vi "IMU Orient Demo.vi"() -> ()   [LabVIEW 2014]
doc: "This example shows how to move a motor connected to an encoder and a wheel, and then read information about the system from an encoder.\n\nThis is an example of how to use feedback (from the encoder) to create an open loop system. If some control method was used, for example using PID, a closed loop system could be created."
uses:
  <vilib>/Rock Robotics/SystemInterfaces/i2clib/i2c_bus.ctl
  <vilib>/Platform/TimedLoop/XDataNode/timing_clust.ctl
  <vilib>/Platform/TimedLoop/XDataNode/nitl_modes.ctl
  <vilib>/Platform/TimedLoop/XDataNode/wakeup.ctl
  <vilib>/Rock Robotics/Network Tables/SD Write Number.vi
  <vilib>/platform/TimedLoop/XDataNode/XDataNode.xnode
  <vilib>/Platform/TimedLoop/XDataNode/XDNodeRunTimeDep.lvlib
panel:
  in  "Status delay":i32=30
  out "Bad result":bool
  in  "Op Mode":T1(ring)=enum."NDOF_FMC_OFF"
  in  "Earth Field (uT)":cluster{"Earth":dbl, "Tolerance":dbl}={"Earth"=51.0, "Tolerance"=5.0}
  out "Anomaly":bool
  out "Z Mag":dbl
  out "Y Mag":dbl
  out "X Mag":dbl
  in  "Read Enable":T2={"Cal Status"=TRUE, "Orientation"=TRUE, "Gyro"=FALSE, "Accelerometer"=FALSE, "Quaternion"=FALSE, "Accel Mode"=enum."Linear", "Magnetometer"=FALSE}
  in  "Calibrate?":bool
  in  "Stored Cal File":string="BNO055 Cal MC P3 11-28-2015 145653"
  out "Q Z":dbl
  out "Q Y":dbl
  out "Q X":dbl
  out "Q W":dbl
  out "GR X":dbl
  out "GR Y":dbl
  out "GR Z":dbl
  in  "Gyro Reset":bool
  out "A X":dbl
  out "A Y":dbl
  out "A Z":dbl
  out "G X":dbl(graph)
  out "G Y":dbl(graph)
  out "G Z":dbl(graph)
  out "M 2":T3
  out "A 2":T3
  out "G 2":T3
  out "S 2":T3
  out "Pitch":dbl(graph)
  out "Roll":dbl(graph)
  out "Yaw":dbl(graph)
  out "M":T3
  out "A":T3
  out "G":T3
  out "S":T3
  in  "I2C Bus":T4=enum."I2C MXP"
  in  "Period (dt in ms)":i64=20
  out "Late?":bool
  # "Magnetic Field Strength (uT)"
  # "Acceleration (mG)"
  # "Gyro Rate (Degrees per Second)"
  # "Quaternions"
  # "Cal Status @ Open"
  # "Current Cal Status"
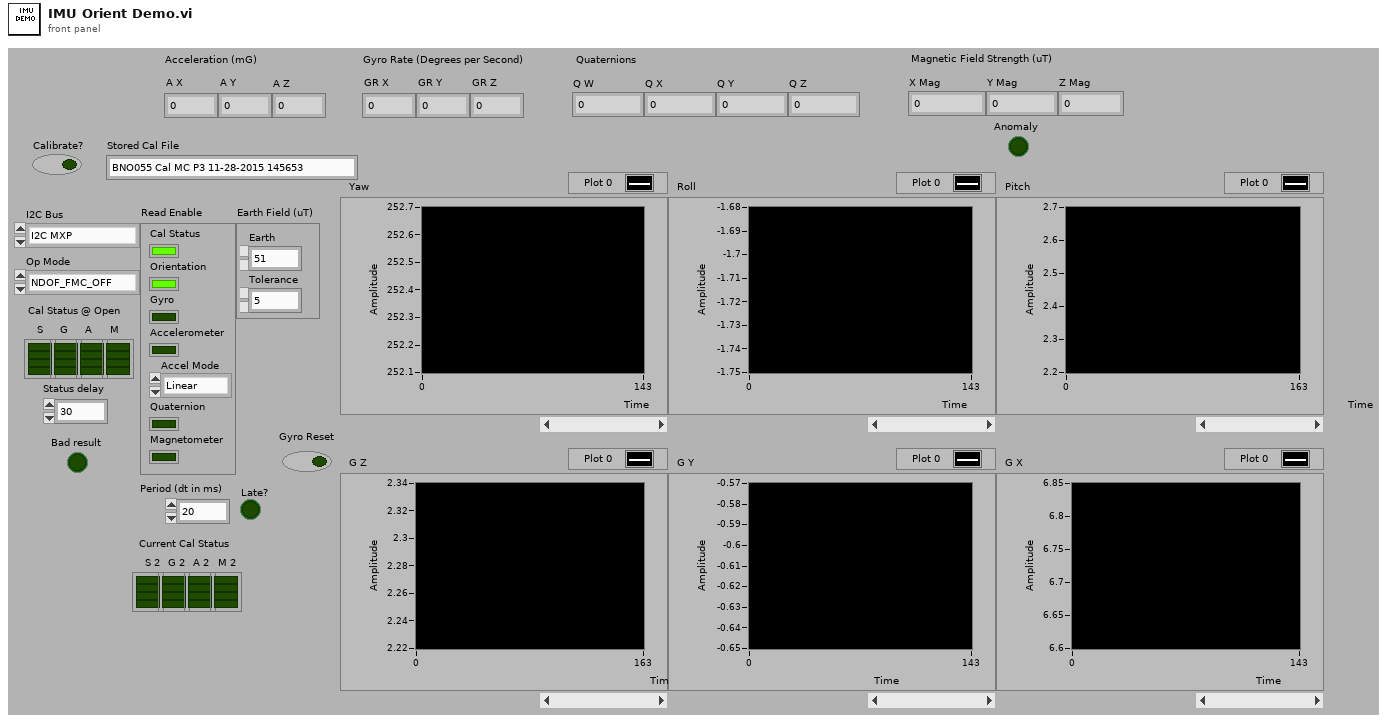
[diagram p1: front panel]
types:
  T1 = enum8{"ConfigMode", "AccOnly", "MagOnly", "GyroOnly", "AccMag", "AccGyro", "MagGyro", "AMG", "IMU", "Compass", "M4G", "NDOF_FMC_OFF", "NDOF"}
  T2 = cluster{"Cal Status":bool, "Orientation":bool, "Gyro":bool, "Accelerometer":bool, "Quaternion":bool, "Accel Mode":enum8{"Raw Data", "Linear", "Gravity"}, "Magnetometer":bool}
  T3 = cluster{"Boolean":bool, "Boolean 2":bool, "Boolean 3":bool, "Boolean 4":bool}
  T4 = typedef "i2c_bus.ctl" = enum16{"I2C On-Board", "I2C MXP", "Invalid"}
  T5 = enum32{"P0", "P1", "P2", "P3", "P4", "P5", "P6", "P7"}
  T6 = cluster{"Cluster":cluster{"[0]":bool, "[1]":bool, "[2]":bool, "[3]":bool}, "Cluster":cluster{"[0]":bool, "[1]":bool, "[2]":bool, "[3]":bool}, "Cluster":cluster{"[0]":bool, "[1]":bool, "[2]":bool, "[3]":bool}, "Cluster":cluster{"[0]":bool, "[1]":bool, "[2]":bool, "[3]":bool}}
  T7 = typedef "WPI_I2CDevRef.ctl" = cluster{"DevStatus":errorcluster, "Controller":T8, "Device Address":u8, "Handle":i32, "I2C Bus":T4}
  T8 = typedef "FPGA_TypedefDigitalModule.ctl" = enum16{"Controller 1"}
  T9 = cluster{"[0]":bool, "[1]":bool, "[2]":bool, "[3]":bool}
  T10 = typedef "XDNodeRunTimeDep.lvlib/timing_clust.ctl" = cluster{"Expected End [f-1]":u64, "Actual End [f-1]":u64, "Finished Late? [f-1]":bool, "Expected End [i-1]":u64, "Actual End [i-1]":u64, "Finished Late? [i-1]":bool, "Expected Start [i]":u64, "Actual Start [i]":u64, "Expected Start [f]":u64, "Actual Start [f]":u64, "Source Name":string, "Structure Name":string, "Period":i64, "Deadline":i64, "Offset":i64, "Start":i64, "Priority":i32, "Timeout":i32, "Mode":T11, "Wakeup Reason":T12, "Error":errorcluster, "Source Type":string, "Secondary Source Type":string, "Global End Time":u64, "Global Start Time":u64, "Frame Duration":u64, "Iteration Duration":u64, "Assigned CPU":i32, "I/O Scan Engine Mode":u32}
  T11 = typedef "XDNodeRunTimeDep.lvlib/nitl_modes.ctl" = enum32{"No Change", "Process missed periods, maintain original phase", "Discard missed periods, maintain original phase", "Process missed periods, ignore original phase", "Discard missed periods, ignore original phase"}
  T12 = typedef "XDNodeRunTimeDep.lvlib/wakeup.ctl" = enum32{"Normal", "Aborted", "Asynchronous wakeup", "Timing source error", "Timed loop error", "Timeout"}
  T13 = cluster{"Mag":cluster{"[0]":bool, "[1]":bool, "[2]":bool, "[3]":bool}, "Acc":cluster{"[0]":bool, "[1]":bool, "[2]":bool, "[3]":bool}, "Gyro":cluster{"[0]":bool, "[1]":bool, "[2]":bool, "[3]":bool}, "Sys":cluster{"[0]":bool, "[1]":bool, "[2]":bool, "[3]":bool}}
  T14 = cluster{"X Gyro":dbl, "Y Gyro":dbl, "Z Gyro":dbl, "X Rate":dbl, "Y Rate":dbl, "Z Rate":dbl}
  T15 = cluster{"X Mag":dbl, "Y Mag":dbl, "Z Mag":dbl, "Anomaly":bool}
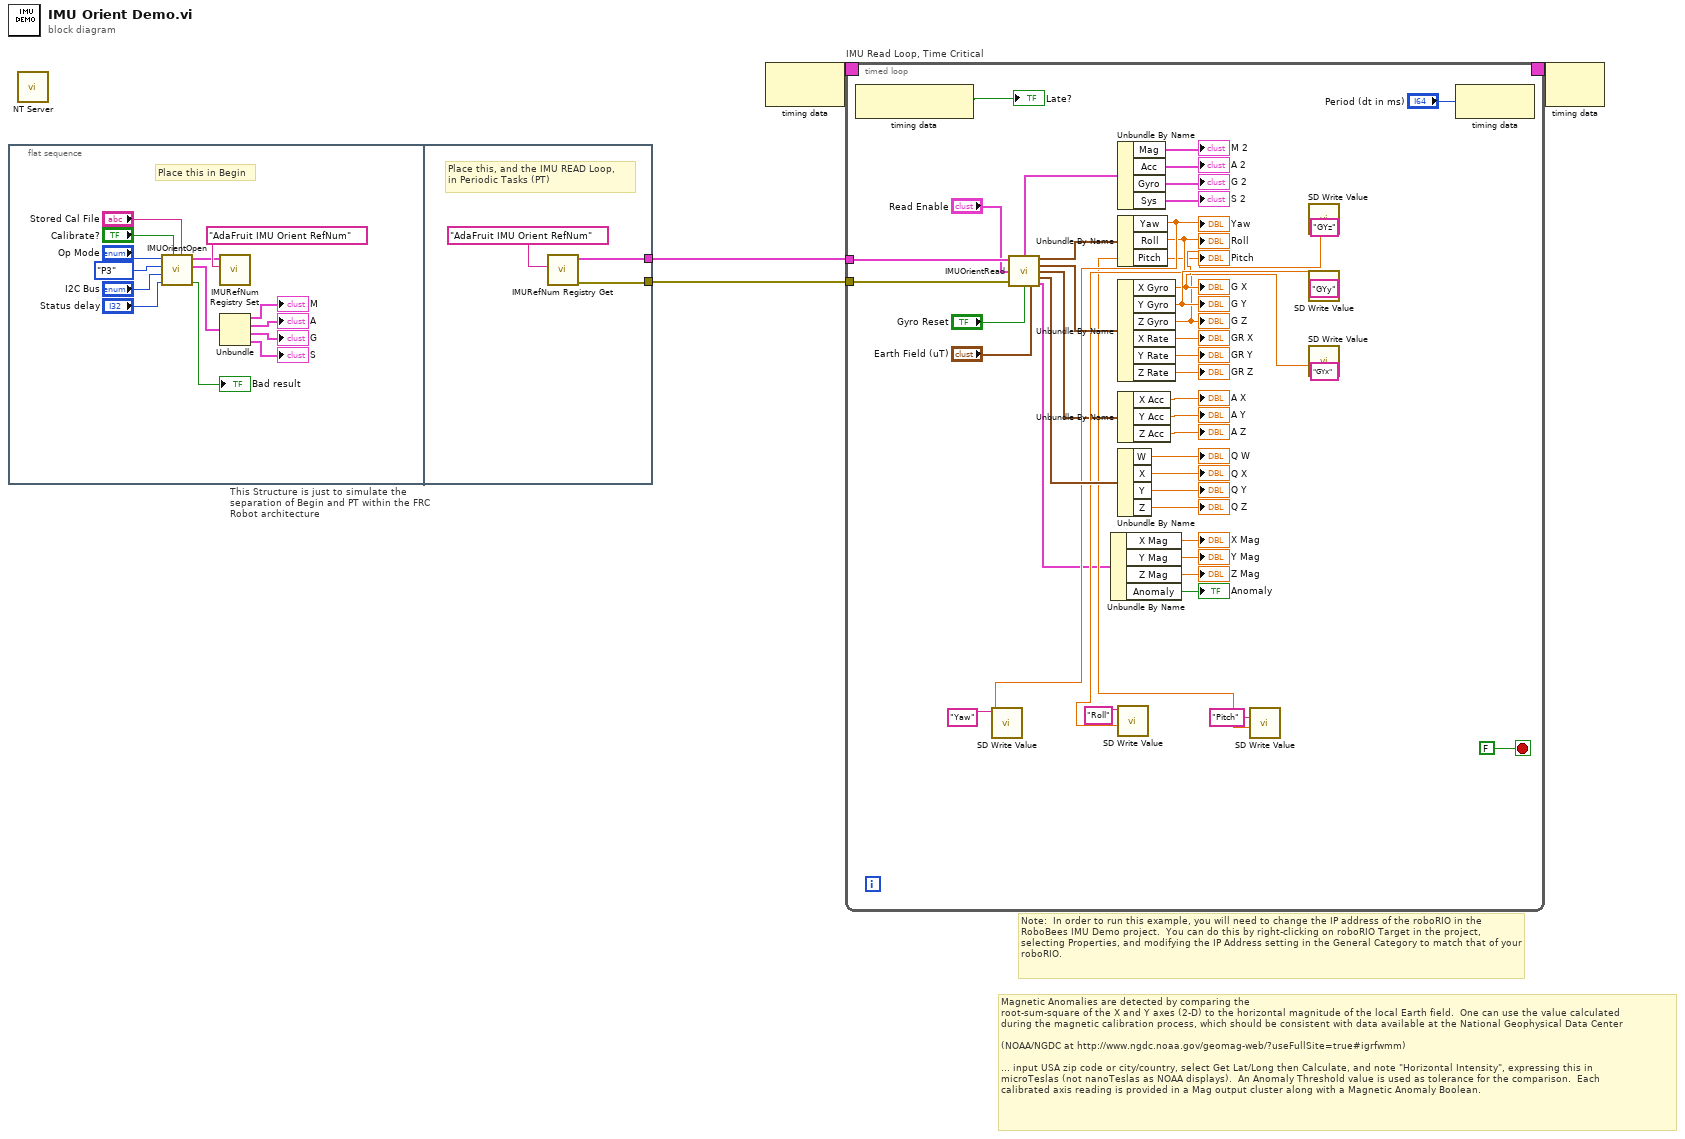
[diagram p0: block diagram]
diagram:
  # "Magnetic Anomalies are detected by comparing the\nroot-sum-square of the X and Y axes (2-D) to the horizontal magnitude of the local Earth field.  One can use the value calculated\nduring the magnetic calibration process, which should be consistent with data available at the National Geophysical Data Center\n\n(NOAA/NGDC at http://www.ngdc.noaa.gov/geomag-web/?useFullSite=true#igrfwmm)\n\n... input USA zip code or city/country, select Get Lat/Long then Calculate, and note \"Horizontal Intensity\", expressing this in\nmicroTeslas (not nanoTeslas as NOAA displays).  An Anomaly Threshold value is used as tolerance for the comparison.  Each\ncalibrated axis reading is provided in a Mag output cluster along with a Magnetic Anomaly Boolean."
  # "Note:  In order to run this example, you will need to change the IP address of the roboRIO in the RoboBees IMU Demo project.  You can do this by right-clicking on roboRIO Target in the project, selecting Properties, and modifying the IP Address setting in the General Category to match that of your roboRIO."
  n1 = flat-sequence "This Structure is just to simulate the separation of Begin and PT within the FRC Robot architecture" {
    tunnel: [w21] -> w1
    tunnel: [w20] -> w4
    frame #0 {
      # "Place this in Begin"
      n2 = call "IMUOrientOpen.vi"("Stored Cal File"="Stored Cal File", "Calibrate?"="Calibrate?", "Status delay"="Status delay", "I2C Bus 2"="I2C Bus", "Placement"=T5."P3", "Op Mode"="Op Mode") -> ("Bad result"=→"Bad result":bool, "Cal Status"=w10:T6, "I2CDevRef"=w9:T7)  [unwired: 3 in]
      n3 = call "IMURefNum Registry Set.vi"("refnum name"="AdaFruit IMU Orient RefNum", "I2CDevRef in"=w9) -> ()  [unwired: 8 in, 2 out]
      n4 = Unbundle(w10) -> ("Cluster"=→"M":T9, "Cluster"=→"A":T9, "Cluster"=→"G":T9, "Cluster"=→"S":T9)
    }
    frame #1 {
      # "Place this, and the IMU READ Loop,\nin Periodic Tasks (PT)"
      n5 = call "IMURefNum Registry Get.vi"("refnum name"="AdaFruit IMU Orient RefNum") -> ("error out"=w20:errorcluster, "I2CDevRef out"=w21:T7)  [unwired: 9 in]
    }
  }
  n6 = call <vilib>:"NT Server.vi"() -> ()  [unwired: 12 in]
  n7 = node-c288() -> (w3:T10)  [unwired: 1 in]
  n8 = timed-loop "IMU Read Loop, Time Critical" {
    timing: w3 -> [_]
    timing-out: [_] -> w2
    tunnel: w4 -> [w61]
    tunnel: w1 -> [w62]
    stop <- FALSE stop-if-true
    n9 = node-c288() -> (→"Late?":bool)  [unwired: 1 in]
    n10 = call "IMUOrientRead.vi"("I2CDevRef"=w62, "Read Enable"="Read Enable", "error in"=w61, "Gyro Reset"="Gyro Reset", "Earth Field (uT)"="Earth Field (uT)") -> ("Cal Status"=w60:T13, "Orient Y/R/P"=w35:cluster{"Yaw":dbl, "Roll":dbl, "Pitch":dbl}, "Gyro X,Y,Z"=w38:T14, "Acc X,Y,Z"=w31:cluster{"X Acc":dbl, "Y Acc":dbl, "Z Acc":dbl}, "Quaternions"=w37:cluster{"W":dbl, "X":dbl, "Y":dbl, "Z":dbl}, "Mag Field X,Y,Z"=w27:T15)  [unwired: 5 in]
    n11 = Unbundle By Name(w27) -> ("X Mag"=→"X Mag":dbl, "Y Mag"=→"Y Mag":dbl, "Z Mag"=→"Z Mag":dbl, "Anomaly"=→"Anomaly":bool)
    n12 = Unbundle By Name(w60) -> ("Mag"=→"M 2":T9, "Acc"=→"A 2":T9, "Gyro"=→"G 2":T9, "Sys"=→"S 2":T9)
    n13 = Unbundle By Name(w35) -> ("Yaw"=w34:dbl, "Roll"=w33:dbl, "Pitch"=w32:dbl)
    "Yaw" <- w34
    "Roll" <- w33
    "Pitch" <- w32
    n14 = call-poly <vilib>:"SD Write Value.vi"("Numeric"=w34, "Name"="Yaw") -> ()  [unwired: 8 in, 2 out]
    n15 = Unbundle By Name(w38) -> ("X Gyro"=w44:dbl, "Y Gyro"=w45:dbl, "Z Gyro"=w43:dbl, "X Rate"=→"GR X":dbl, "Y Rate"=→"GR Y":dbl, "Z Rate"=→"GR Z":dbl)
    "G X" <- w44
    "G Y" <- w45
    "G Z" <- w43
    n16 = Unbundle By Name(w31) -> ("X Acc"=→"A X":dbl, "Y Acc"=→"A Y":dbl, "Z Acc"=→"A Z":dbl)
    n17 = Unbundle By Name(w37) -> ("W"=→"Q W":dbl, "X"=→"Q X":dbl, "Y"=→"Q Y":dbl, "Z"=→"Q Z":dbl)
    n18 = call-poly <vilib>:"SD Write Value.vi"("Numeric"=w33, "Name"="Roll") -> ()  [unwired: 8 in, 2 out]
    n19 = call-poly <vilib>:"SD Write Value.vi"("Numeric"=w32, "Name"="Pitch") -> ()  [unwired: 8 in, 2 out]
    n20 = call-poly <vilib>:"SD Write Value.vi"("Numeric"=w44, "Name"="GYz") -> ()  [unwired: 8 in, 2 out]
    n21 = call-poly <vilib>:"SD Write Value.vi"("Numeric"=w45, "Name"="GYy") -> ()  [unwired: 8 in, 2 out]
    n22 = call-poly <vilib>:"SD Write Value.vi"("Numeric"=w43, "Name"="GYx") -> ()  [unwired: 8 in, 2 out]
    n23 = node-c288("Period (dt in ms)") -> ()  [unwired: 1 out]
  }
  n24 = node-c288(w2) -> ()  [unwired: 1 out]
